vi "Mining and Dumping_r4.vi"() -> ()   [LabVIEW 2015]
uses:
  <vilib>/myRIO/Instrument Drivers/Onboard IO/PWM/typedefs/PWM Reference.ctl
  <vilib>/myRIO/Common/Instrument Driver Framework/Utilities/typedefs/myRIO Generic Hardware Reference.ctl
  <vilib>/myRIO/Common/Instrument Driver Framework/Utilities/typedefs/Hardware Version Enum.ctl
  <vilib>/myRIO/Common/Instrument Driver Framework/Utilities/typedefs/myRIO v1.0 Reference.ctl
  <vilib>/myRIO/Common/Instrument Driver Framework/Utilities/typedefs/Generic FPGA Reference.ctl
  <vilib>/myRIO/Common/Instrument Driver Framework/myRIO v1.0/PWM/typedefs/PWM Channels Enum.ctl
  <vilib>/myRIO/Instrument Drivers/Onboard IO/PWM/typedefs/PWM Configuration.ctl
  <vilib>/userdefined/High Color/nirio_resource_hc.ctl
  <vilib>/myRIO/Instrument Drivers/Onboard IO/AI/typedefs/AI Reference.ctl
  <vilib>/myRIO/Common/Instrument Driver Framework/myRIO v1.0/AI/typedefs/AI Channels List.ctl
  <vilib>/myRIO/Common/Instrument Driver Framework/myRIO v1.0/AI/typedefs/AI Channels Enum.ctl
  <vilib>/myRIO/Common/Instrument Driver Framework/Utilities/typedefs/Analog Scaling Constants List.ctl
  <vilib>/myRIO/Common/Instrument Driver Framework/Utilities/typedefs/Analog Scaling Constants.ctl
  <vilib>/myRIO/Common/Instrument Driver Framework/Utilities/vis/Is FPGA Ref Available.vi
  <vilib>/myRIO/Common/Instrument Driver Framework/myRIO v1.0/PWM/vis/myRIO v1.1 Open PWM.vi
  <vilib>/myRIO/Instrument Drivers/Onboard IO/PWM/vis/Set Duty Cycle and Frequency.vi
  <vilib>/myRIO/Common/Instrument Driver Framework/myRIO v1.0/AI/vis/myRIO v1.1 Open AI.vi
  <vilib>/myRIO/Instrument Drivers/Onboard IO/AI/vis/Read.vi
  <vilib>/myRIO/Common/Instrument Driver Framework/Utilities/vis/Validate Channels.vi
  <vilib>/myRIO/Common/Instrument Driver Framework/myRIO v1.0/PWM/vis/myRIO v1.0 Reserve PWM.vi
  <vilib>/myRIO/Common/Instrument Driver Framework/myRIO v1.0/AI/vis/myRIO v1.0 Reserve AI.vi
  <vilib>/myRIO/Common/Instrument Driver Framework/myRIO v1.0/PWM/vis/myRIO v1.0 Build MUX Configuration PWM.vi
  <vilib>/myRIO/Common/Instrument Driver Framework/myRIO v1.0/Resource Manager/vis/myRIO v1.0 Reserve Channel List.vi
  <vilib>/myRIO/Common/Instrument Driver Framework/myRIO v1.0/AI/vis/myRIO v1.0 Build MUX Configuration AI.vi
  <vilib>/myRIO/Common/Instrument Driver Framework/myRIO v1.0/Resource Manager/vis/myRIO v1.0 Create Configuration List.vi
  <vilib>/myRIO/Common/Instrument Driver Framework/myRIO v1.0/Resource Manager/vis/myRIO v1.0 Reserve Channel.vi
  <vilib>/myRIO/Common/Instrument Driver Framework/myRIO v1.0/Resource Manager/vis/myRIO v1.0 Unreserve Channel.vi
  <vilib>/myRIO/Common/Instrument Driver Framework/myRIO v1.0/Resource Manager/vis/myRIO v1.0 Build Mutex Name.vi
  <vilib>/Utility/VariantDataType/GetNumericInfo.vi
  <vilib>/Utility/error.llb/Error Cluster From Error Code.vi
  <vilib>/myRIO/Common/Instrument Driver Framework/myRIO v1.0/myRIO v1.1 Open.vi
  <vilib>/myRIO/Common/Instrument Driver Framework/Utilities/vis/IO Manager.vi
  <vilib>/myRIO/Common/Instrument Driver Framework/Utilities/vis/Configuration Manager.vi
  <vilib>/myRIO/Common/Instrument Driver Framework/myRIO v1.0/Resource Manager/vis/myRIO v1.0 Configure IO.vi
  <vilib>/myRIO/Common/Instrument Driver Framework/myRIO v1.0/myRIO v1.0 Close.vi
  <vilib>/myRIO/Common/Instrument Driver Framework/myRIO v1.0/PWM/vis/myRIO v1.0 Write PWM.vi
  <vilib>/myRIO/Common/Instrument Driver Framework/myRIO v1.0/AI/vis/myRIO v1.0 Get Scaling Constants AI.vi
  <vilib>/myRIO/Common/Instrument Driver Framework/myRIO v1.0/AI/vis/myRIO v1.0 Read AI.vi
  <vilib>/myRIO/Express VI/Onboard IO/PWM/PWM Express VI.xnode
  <vilib>/myRIO/Instrument Drivers/Onboard IO/PWM/vis/myRIO PWM Open.xnode
  <vilib>/myRIO/Express VI/Onboard IO/AI/AI Express VI.xnode
  <vilib>/myRIO/Instrument Drivers/Onboard IO/AI/vis/myRIO AI Open.xnode
  <vilib>/myRIO/Instrument Drivers/Onboard IO/PWM/PWM.lvlib
  <vilib>/myRIO/Instrument Drivers/Onboard IO/AI/AI.lvlib
panel:
  out "unjammed":bool
  in  "Mine or Dump":i16
  out "Stop Dumping":bool
  in  "Stop":bool
  out "Servo Positioin 2":dbl
  out "Servo Position 1":dbl
  out "Servo Stop":i64
  out "Stop Mining":bool
  out "Full":bool
  # "0=Idle\n1=Mine\n-1=Dump"
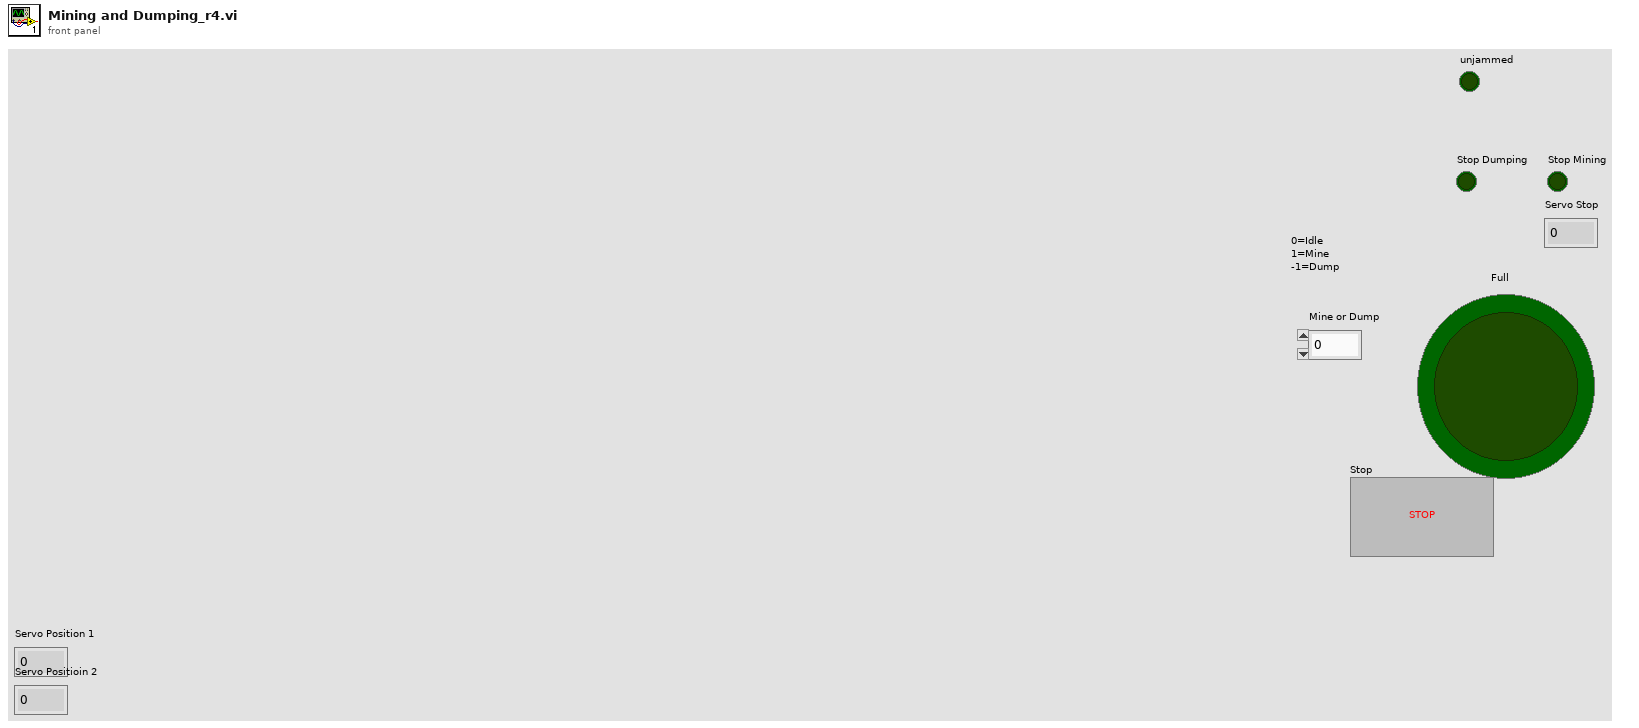
[diagram p1: front panel]
types:
  T1 = typedef "PWM.lvlib/PWM Reference.ctl" = cluster{"myRIO Reference":T2, "PWM Channels Enum":T6, "PWM Configuration":T7}
  T2 = typedef "myRIO Generic Hardware Reference.ctl" = cluster{"myRIO Model":T3, "myRIO Hardware Reference":T4}
  T3 = typedef "Hardware Version Enum.ctl" = enum16{"Unknown", "myRIO-1900", "myRIO-1950", "roboRIO"}
  T4 = typedef "myRIO v1.0 Reference.ctl" = cluster{"Generic FPGA Reference":T5, "Allow multiple opens":bool}
  T5 = typedef "Generic FPGA Reference.ctl" = refnum<k20>
  T6 = typedef "PWM Channels Enum.ctl" = enum16{"Not Connected", "C/PWM0", "C/PWM1", "A/PWM0", "A/PWM1", "A/PWM2", "B/PWM0", "B/PWM1", "B/PWM2", "PWM/PWM0", "PWM/PWM1", "PWM/PWM2", "PWM/PWM3", "PWM/PWM4", "PWM/PWM5", "PWM/PWM6", "PWM/PWM7", "PWM/PWM8", "PWM/PWM9"}
  T7 = typedef "PWM.lvlib/PWM Configuration.ctl" = cluster{"Frequency":dbl, "Duty Cycle":dbl}
  T8 = typedef "nirio_resource_hc.ctl" = tag
  T9 = typedef "AI.lvlib/AI Reference.ctl" = cluster{"myRIO Reference":T2, "AI Channels List":T10, "AI Scaling Constants List":T12}
  T10 = typedef "AI Channels List.ctl" = T11[]
  T11 = typedef "AI Channels Enum.ctl" = enum16{"Not Connected", "AudioIn/Left", "AudioIn/Right", "C/AI0", "C/AI1", "A/AI0", "A/AI1", "A/AI2", "A/AI3", "B/AI0", "B/AI1", "B/AI2", "B/AI3", "AI/AI0", "AI/AI1", "AI/AI2", "AI/AI3"}
  T12 = typedef "Analog Scaling Constants List.ctl" = T13[]
  T13 = typedef "Analog Scaling Constants.ctl" = cluster{"LSB Weight (Volts)":dbl, "Offset (Volts)":dbl, "Signed?":bool}
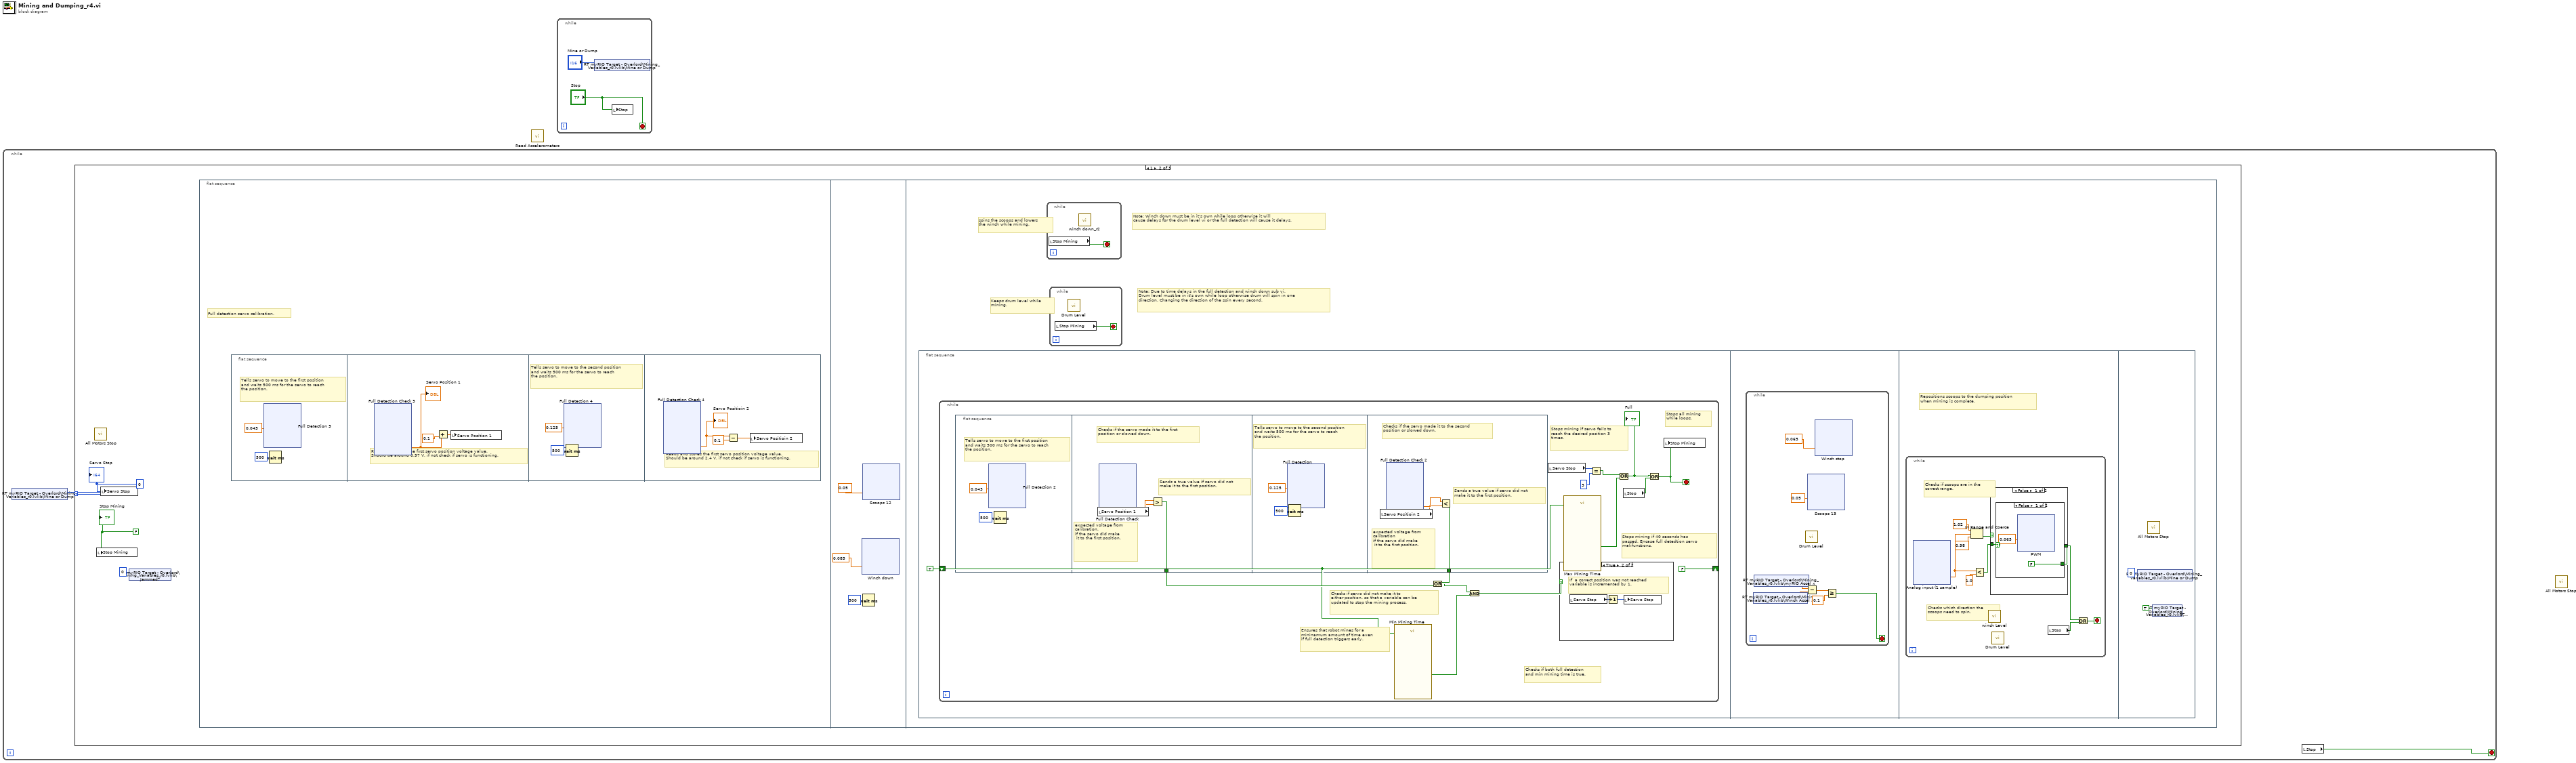
[diagram p0: block diagram]
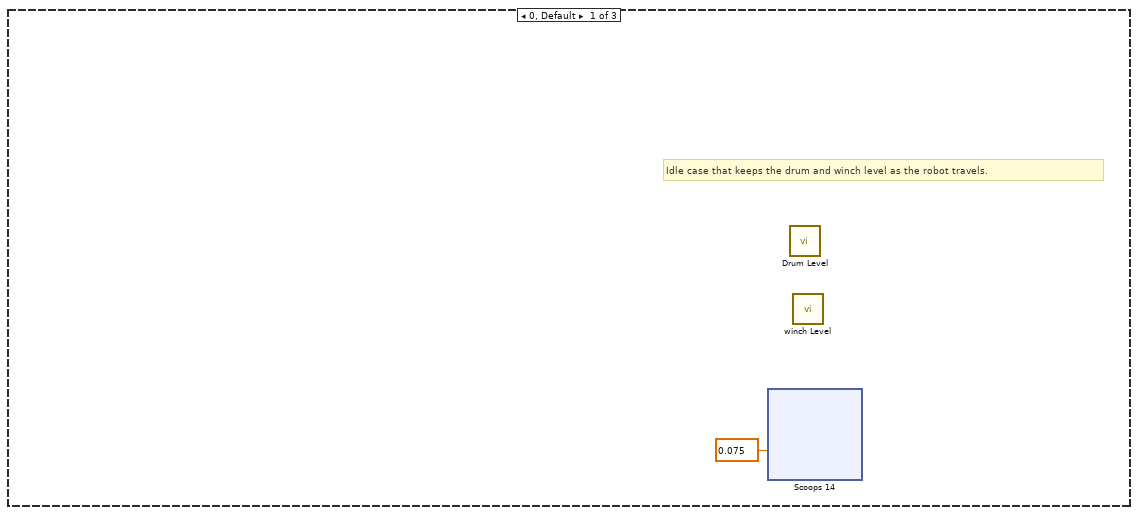
[diagram p2: hidden frame]
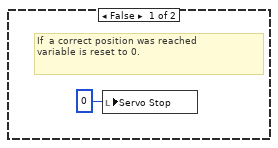
[diagram p3: hidden frame]
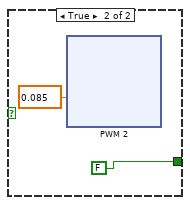
[diagram p4: hidden frame]
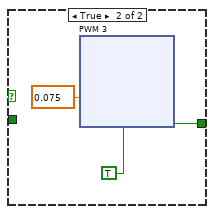
[diagram p5: hidden frame]
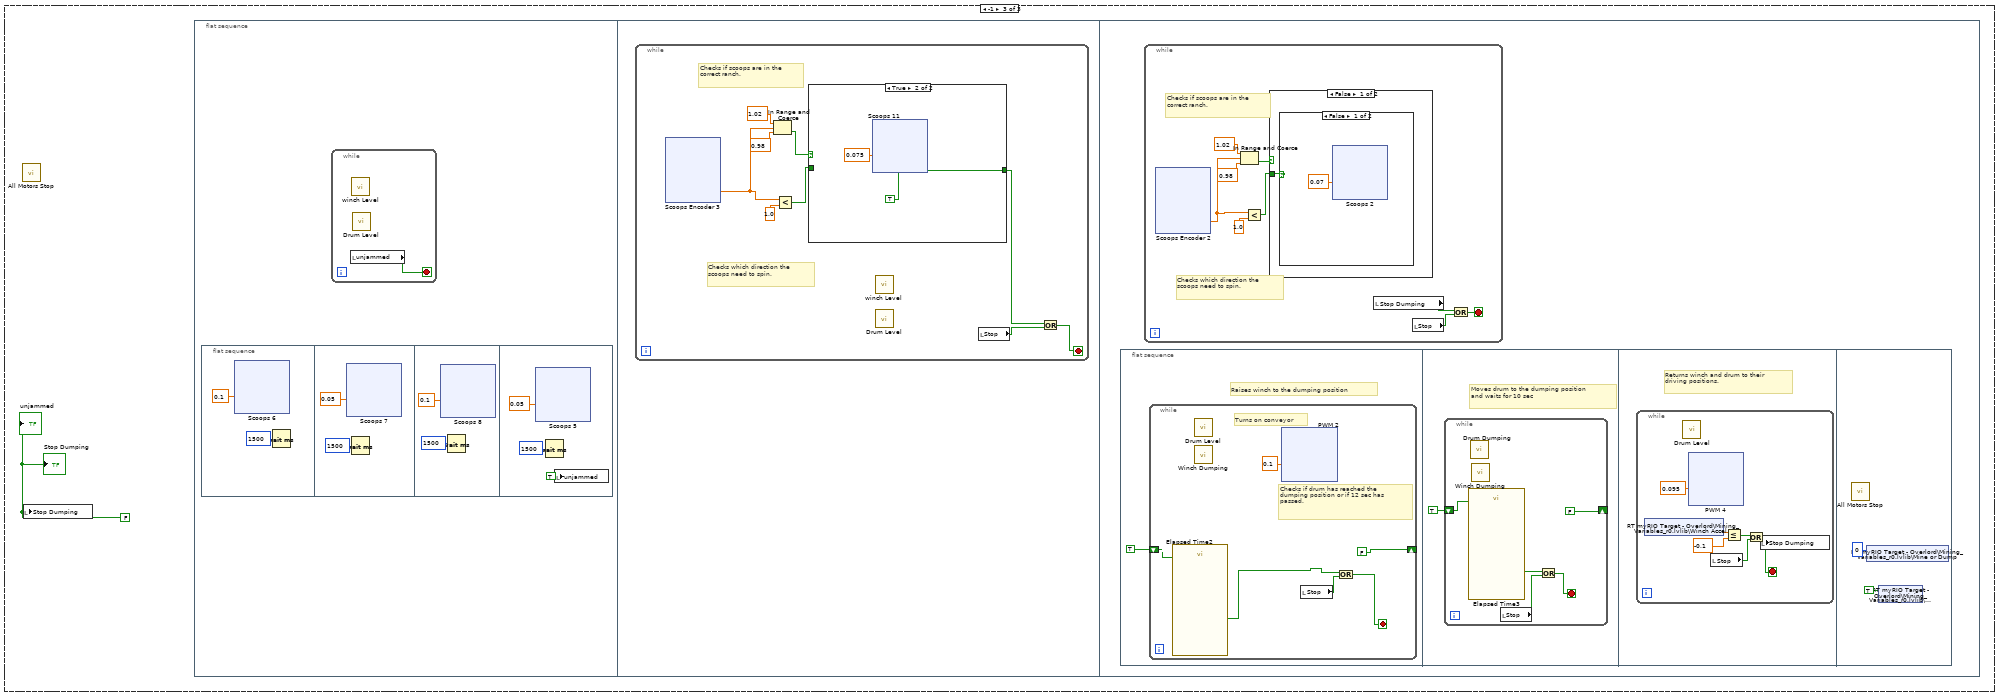
[diagram p6: hidden frame]
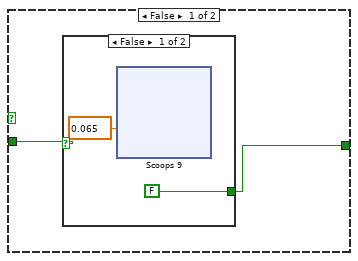
[diagram p7: hidden frame]
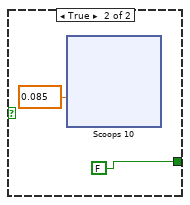
[diagram p8: hidden frame]
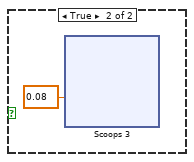
[diagram p9: hidden frame]
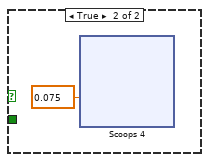
[diagram p10: hidden frame]
diagram:
  n1 = while {
    stop <- w1 stop-if-true
    n2 = shared-variable "RT myRIO Target - Overlord\\Mining_Variables_r0.lvlib\\Mine or Dump"() -> (w2:i16)  [unwired: 1 in, 1 out]
    n3 = case shown="1" w2 {
      frame 0, Default {
        # "Idle case that keeps the drum and winch level as the robot travels."
        n4 = xnode "Scoops 14"("Duty Cycle"=0.075) -> ()  [unwired: 1 in, 1 out]
        n5 = call "Drum Level.vi"() -> ()  [unwired: 12 in]
        n6 = call "winch Level.vi"() -> ()  [unwired: 12 in]
      }
      frame 1 {
        w41 = FALSE ("Stop")
        w40 = i64 0 ("Servo Stop")
        n7 = call "All Motors Stop.vi"() -> ()  [unwired: 12 in]
        n8 = local write "Stop Mining"(w41) -> ()
        n9 = local write "Servo Stop"(w40) -> ()
        n10 = shared-variable "RT myRIO Target - Overlord\\Mining_Variables_r0.lvlib\\Jammed?"(u16 0 ("Jammed?")) -> ()  [unwired: 1 in, 1 out]
        n11 = flat-sequence {
          frame #0 {
            # "Full detection servo calibration."
            n12 = flat-sequence {
              frame #0 {
                # "Tells servo to move to the first position\nand waits 500 ms for the servo to reach \nthe position."
                n13 = xnode "Full Detection 3"("Duty Cycle"=0.043) -> ()  [unwired: 1 in, 1 out]
                n14 = Wait (ms)(milliseconds to wait=u32 500) -> ()  [unwired: 1 out]
              }
              frame #1 {
                # "Reads and stores the first servo position voltage value. \nShould be around 0.97 V. if not check if servo is functioning."
                n15 = xnode "Full Detection Check 3"() -> ("A/AI0 (Pin 3)"=w80:dbl)  [unwired: 1 in, 1 out]
                "Servo Position 1" <- w80
                n16 = Add(x=w80, y=0.1) -> (x+y=w81:dbl)
                n17 = local write "Servo Position 1"(w81) -> ()
              }
              frame #2 {
                # "Tells servo to move to the second position\nand waits 500 ms for the servo to reach \nthe position."
                n18 = xnode "Full Detection 4"("Duty Cycle"=0.125) -> ()  [unwired: 1 in, 1 out]
                n19 = Wait (ms)(milliseconds to wait=u32 500) -> ()  [unwired: 1 out]
              }
              frame #3 {
                # "Reads and stores the first servo position voltage value. \nShould be around 2.4 V. if not check if servo is functioning."
                n20 = xnode "Full Detection Check 4"() -> ("A/AI0 (Pin 3)"=w157:dbl)  [unwired: 1 in, 1 out]
                "Servo Positioin 2" <- w157
                n21 = Subtract(x=w157, y=0.1) -> (x-y=w158:dbl)
                n22 = local write "Servo Positioin 2"(w158) -> ()
              }
            }
          }
          frame #1 {
            n23 = xnode "Winch down"("Duty Cycle"=0.085) -> ()  [unwired: 1 in, 1 out]
            n24 = xnode "Scoops 12"("Duty Cycle"=0.05) -> ()  [unwired: 1 in, 1 out]
            n25 = Wait (ms)(milliseconds to wait=u32 500) -> ()  [unwired: 1 out]
          }
          frame #2 {
            # "Note: Winch down must be in it's own while loop otherwise it will \ncause delays for the drum level vi or the full detection will cause it delays."
            # "Note: Due to time delays in the full detection and winch down sub vi.\nDrum level must be in it's own while loop otherwise drum will spin in one\ndirection. Changing the direction of the spin every second."
            # "spins the scoops and lowers\nthe winch while mining."
            # "Keeps drum level while \nmining."
            n26 = flat-sequence {
              frame #0 {
                n27 = while {
                  shift-right: [FALSE] -> _
                  shift-left: TRUE -> [w271]
                  stop <- w274 stop-if-true
                  # "Stops all mining \nwhile loops."
                  # "Stops mining if 40 seconds has \npassed. Encase full detedtion servo \nmalifunctions."
                  # "Stops mining if servo fails to \nreach the desired position 3\ntimes."
                  # "Checks if both full detection \nand min mining time is true."
                  # "Ensures that robot mines for a \nmininamum amount of time even\nif full detection triggers early."
                  # "Checks if servo did not make it to\neither position. so that a variable can be \nupdated to stop the mining process."
                  n28 = flat-sequence {
                    tunnel: [w327] -> w283
                    tunnel: [w403] -> w284
                    frame #0 {
                      # "Tells servo to move to the first position\nand waits 500 ms for the servo to reach \nthe position."
                      n29 = xnode "Full Detection 2"("Duty Cycle"=0.043) -> ()  [unwired: 1 in, 1 out]
                      n30 = Wait (ms)(milliseconds to wait=u32 500) -> ()  [unwired: 1 out]
                    }
                    frame #1 {
                      # "Sends a true value if servo did not \nmake it to the first position."
                      # "expected voltage from \ncalibration.\nif the servo did make\n it to the first position."
                      # "Checks if the servo made it to the first \nposition or slowed down."
                      n31 = local read "Servo Position 1"() -> (w325:dbl)
                      n32 = xnode "Full Detection Check"() -> ("A/AI0 (Pin 3)"=w326:dbl)  [unwired: 1 in, 1 out]
                      n33 = Greater?(x=w326, y=w325) -> (0:w327:bool)
                    }
                    frame #2 {
                      # "Tells servo to move to the second position\nand waits 500 ms for the servo to reach \nthe position."
                      n34 = xnode "Full Detection"("Duty Cycle"=0.125) -> ()  [unwired: 1 in, 1 out]
                      n35 = Wait (ms)(milliseconds to wait=u32 500) -> ()  [unwired: 1 out]
                    }
                    frame #3 {
                      # "Sends a true value if servo did not \nmake it to the first position."
                      # "expected voltage from \ncalibration\nif the servo did make\n it to the first position."
                      # "Checks if the servo made it to the second \nposition or slowed down."
                      n36 = local read "Servo Positioin 2"() -> (w402:dbl)
                      n37 = xnode "Full Detection Check 2"() -> ("A/AI0 (Pin 3)"=w404:dbl)  [unwired: 1 in, 1 out]
                      n38 = Less?(x=w404, y=w402) -> (x < y?=w403:bool)
                    }
                  }
                  n39 = call "Min Mining Time"("Reset"=w271) -> ("Time has Elapsed"=w276:bool)  [unwired: 11 in, 7 out]
                  n40 = Or(x=w284, y=w283) -> (x .or. y?=w277:bool)
                  n41 = And(x=w277, y=w276) -> (x .and. y?=w278:bool)
                  n42 = local read "Servo Stop"() -> (w281:i64)
                  n43 = case shown="True" w278 {
                    frame False {
                      # "If  a correct position was reached \nvariable is reset to 0."
                      n44 = local write "Servo Stop"(i64 0 ("Servo Stop")) -> ()
                    }
                    frame True {
                      # "If  a correct position was not reached \nvariable is incremented by 1."
                      n45 = local read "Servo Stop"() -> (w287:i64)
                      n46 = Increment(x=w287) -> (x+1=w286:i64)
                      n47 = local write "Servo Stop"(w286) -> ()
                    }
                  }
                  n48 = call "Max Mining Time"("Reset"=w271) -> ("Time has Elapsed"=w280:bool)  [unwired: 11 in, 7 out]
                  n49 = Equal?(x=w281, y=i64 3) -> (x = y?=w279:bool)
                  n50 = Or(x=w279, y=w280) -> (x .or. y?=w275:bool)
                  "Full" <- w275
                  n51 = local read "Stop"() -> (w273:bool)
                  n52 = Or(x=w275, y=w273) -> (x .or. y?=w274:bool)
                  n53 = local write "Stop Mining"(w274) -> ()
                }
              }
              frame #1 {
                n54 = while {
                  stop <- w442 stop-if-true
                  n55 = shared-variable "RT myRIO Target - Overlord\\Mining_Variables_r0.lvlib\\Winch Accel x"() -> (w445:dbl)  [unwired: 1 in, 1 out]
                  n56 = shared-variable "RT myRIO Target - Overlord\\Mining_Variables_r0.lvlib\\myRIO Accel x"() -> (w446:dbl)  [unwired: 1 in, 1 out]
                  n57 = call "Drum Level.vi"() -> ()  [unwired: 12 in]
                  n58 = Subtract(x=w446, y=w445) -> (x-y=w444:dbl)
                  n59 = xnode "Scoops 13"("Duty Cycle"=0.05) -> ()  [unwired: 1 in, 1 out]
                  n60 = xnode "Winch stop"("Duty Cycle"=0.065) -> ()  [unwired: 1 in, 1 out]
                  n61 = Greater Or Equal?(x=w444, y=0.1) -> (x >= y?=w442:bool)
                }
              }
              frame #2 {
                # "Repositions scoops to the dumping position\nwhen mining is complete."
                n62 = while {
                  stop <- w521 stop-if-true
                  # "Checks which direction the \nscoops need to spin."
                  # "Checks if scoops are in the\ncorrect range."
                  n63 = xnode "Analog input (1 sample)"() -> ("A/AI1 (Pin 5)"=w524:dbl)  [unwired: 1 in, 1 out]
                  n64 = In Range and Coerce(upper limit=1.02, x=w524, lower limit=0.98) -> (In Range?=w525:bool)  [unwired: 1 out]
                  n65 = Less?(x=w524, y=1.0) -> (x < y?=w526:bool)
                  n66 = call "winch Level.vi"() -> ()  [unwired: 12 in]
                  n67 = case shown="False" w525 {
                    tunnel: w526 -> [w529 _]
                    tunnel: [w528 TRUE] -> w520
                    frame False {
                      n68 = case shown="False" w529 {
                        tunnel: [FALSE FALSE] -> w528
                        frame False {
                          n69 = xnode "PWM"("Duty Cycle"=0.065) -> ()  [unwired: 1 in, 1 out]
                        }
                        frame True {
                          n70 = xnode "PWM 2"("Duty Cycle"=0.085) -> ()  [unwired: 1 in, 1 out]
                        }
                      }
                    }
                    frame True {
                      n71 = xnode "PWM 3"("Duty Cycle"=0.075) -> ()  [unwired: 1 in, 1 out]
                    }
                  }
                  n72 = call "Drum Level.vi"() -> ()  [unwired: 12 in]
                  n73 = local read "Stop"() -> (w519:bool)
                  n74 = Or(x=w520, y=w519) -> (x .or. y?=w521:bool)
                }
              }
              frame #3 {
                n75 = shared-variable "RT myRIO Target - Overlord\\Mining_Variables_r0.lvlib\\Mine or Dump"(i16 0 ("Mine or Dump")) -> ()  [unwired: 1 in, 1 out]
                n76 = call "All Motors Stop.vi"() -> ()  [unwired: 12 in]
                n77 = shared-variable "RT myRIO Target - Overlord\\Mining_Variables_r0.lvlib\\Stop"(TRUE ("Stop")) -> ()  [unwired: 1 in, 1 out]
              }
            }
            n78 = while {
              stop <- w269 stop-if-true
              n79 = local read "Stop Mining"() -> (w269:bool)
              n80 = call "winch down_r2.vi"() -> ()  [unwired: 12 in]
            }
            n81 = while {
              stop <- w680 stop-if-true
              n82 = local read "Stop Mining"() -> (w680:bool)
              n83 = call "Drum Level.vi"() -> ()  [unwired: 12 in]
            }
          }
        }
        "Stop Mining" <- w41
        "Servo Stop" <- w40
      }
      frame -1 {
        w681 = FALSE
        n84 = call "All Motors Stop.vi"() -> ()  [unwired: 12 in]
        n85 = local write "Stop Dumping"(w681) -> ()
        n86 = flat-sequence {
          frame #0 {
            n87 = flat-sequence {
              frame #0 {
                n88 = xnode "Scoops 6"("Duty Cycle"=0.1) -> ()  [unwired: 1 in, 1 out]
                n89 = Wait (ms)(milliseconds to wait=u32 1500) -> ()  [unwired: 1 out]
              }
              frame #1 {
                n90 = xnode "Scoops 7"("Duty Cycle"=0.05) -> ()  [unwired: 1 in, 1 out]
                n91 = Wait (ms)(milliseconds to wait=u32 1500) -> ()  [unwired: 1 out]
              }
              frame #2 {
                n92 = xnode "Scoops 8"("Duty Cycle"=0.1) -> ()  [unwired: 1 in, 1 out]
                n93 = Wait (ms)(milliseconds to wait=u32 1500) -> ()  [unwired: 1 out]
              }
              frame #3 {
                n94 = xnode "Scoops 5"("Duty Cycle"=0.05) -> ()  [unwired: 1 in, 1 out]
                n95 = Wait (ms)(milliseconds to wait=u32 1500) -> ()  [unwired: 1 out]
                n96 = local write "unjammed"(TRUE ("unjammed")) -> ()
              }
            }
            n97 = while {
              stop <- w682 stop-if-true
              n98 = local read "unjammed"() -> (w682:bool)
              n99 = call "winch Level.vi"() -> ()  [unwired: 12 in]
              n100 = call "Drum Level.vi"() -> ()  [unwired: 12 in]
            }
          }
          frame #1 {
            n101 = while {
              stop <- w834 stop-if-true
              # "Checks which direction the \nscoops need to spin."
              # "Checks if scoops are in the\ncorrect ranch."
              n102 = xnode "Scoops Encoder 3"() -> ("A/AI1 (Pin 5)"=w837:dbl)  [unwired: 1 in, 1 out]
              n103 = In Range and Coerce(upper limit=1.02, x=w837, lower limit=0.98) -> (In Range?=w836:bool)  [unwired: 1 out]
              n104 = Less?(x=w837, y=1.0) -> (x < y?=w835:bool)
              n105 = case shown="True" w836 {
                tunnel: w835 -> [w842 _]
                tunnel: [w841 TRUE] -> w833
                frame False {
                  n106 = case shown="False" w842 {
                    tunnel: [FALSE FALSE] -> w841
                    frame False {
                      n107 = xnode "Scoops 9"("Duty Cycle"=0.065) -> ()  [unwired: 1 in, 1 out]
                    }
                    frame True {
                      n108 = xnode "Scoops 10"("Duty Cycle"=0.085) -> ()  [unwired: 1 in, 1 out]
                    }
                  }
                }
                frame True {
                  n109 = xnode "Scoops 11"("Duty Cycle"=0.075) -> ()  [unwired: 1 in, 1 out]
                }
              }
              n110 = call "winch Level.vi"() -> ()  [unwired: 12 in]
              n111 = call "Drum Level.vi"() -> ()  [unwired: 12 in]
              n112 = local read "Stop"() -> (w832:bool)
              n113 = Or(x=w833, y=w832) -> (x .or. y?=w834:bool)
            }
          }
          frame #2 {
            n114 = flat-sequence {
              frame #0 {
                # "Raises winch to the dumping position"
                n115 = while {
                  shift-right: [FALSE ("Reset")] -> _
                  shift-left: TRUE ("Reset") -> [w1148]
                  stop <- w1151 stop-if-true
                  # "Turns on conveyor"
                  # "Checks if drum has reached the \ndumping position or if 12 sec has \npassed."
                  n116 = call "Elapsed Time2"("Reset"=w1148) -> ("Time has Elapsed"=w1147:bool)  [unwired: 11 in, 7 out]
                  n117 = call "Drum Level.vi"() -> ()  [unwired: 12 in]
                  n118 = call "Winch Dumping.vi"() -> ()  [unwired: 12 in]
                  n119 = xnode "PWM 2"("Duty Cycle"=0.1) -> ()  [unwired: 1 in, 1 out]
                  n120 = local read "Stop"() -> (w1150:bool)
                  n121 = Or(x=w1147, y=w1150) -> (x .or. y?=w1151:bool)
                }
              }
              frame #1 {
                # "Moves drum to the dumping position\nand waits for 10 sec"
                n122 = while {
                  shift-right: [FALSE ("Reset")] -> _
                  shift-left: TRUE ("Reset") -> [w1189]
                  stop <- w1193 stop-if-true
                  n123 = call "Elapsed Time3"("Reset"=w1189) -> ("Time has Elapsed"=w1192:bool)  [unwired: 11 in, 7 out]
                  n124 = call "Drum Dumping.vi"() -> ()  [unwired: 12 in]
                  n125 = call "Winch Dumping.vi"() -> ()  [unwired: 12 in]
                  n126 = local read "Stop"() -> (w1191:bool)
                  n127 = Or(x=w1192, y=w1191) -> (x .or. y?=w1193:bool)
                }
              }
              frame #2 {
                # "Returns winch and drum to their \ndriving positions."
                n128 = while {
                  stop <- w1194 stop-if-true
                  n129 = shared-variable "RT myRIO Target - Overlord\\Mining_Variables_r0.lvlib\\Winch Accel x"() -> (w1199:dbl)  [unwired: 1 in, 1 out]
                  n130 = call "Drum Level.vi"() -> ()  [unwired: 12 in]
                  n131 = xnode "PWM 4"("Duty Cycle"=0.095) -> ()  [unwired: 1 in, 1 out]
                  n132 = local read "Stop"() -> (w1195:bool)
                  n133 = Less Or Equal?(x=w1199, y=-0.1) -> (x <= y?=w1196:bool)
                  n134 = Or(x=w1196, y=w1195) -> (x .or. y?=w1194:bool)
                  n135 = local write "Stop Dumping"(w1194) -> ()
                }
              }
              frame #3 {
                n136 = call "All Motors Stop.vi"() -> ()  [unwired: 12 in]
                n137 = shared-variable "RT myRIO Target - Overlord\\Mining_Variables_r0.lvlib\\Mine or Dump"(i16 0 ("Mine or Dump")) -> ()  [unwired: 1 in, 1 out]
                n138 = shared-variable "RT myRIO Target - Overlord\\Mining_Variables_r0.lvlib\\Stop"(TRUE ("Stop")) -> ()  [unwired: 1 in, 1 out]
              }
            }
            n139 = while {
              stop <- w993 stop-if-true
              # "Checks which direction the \nscoops need to spin."
              # "Checks if scoops are in the\ncorrect ranch."
              n140 = xnode "Scoops Encoder 2"() -> ("A/AI1 (Pin 5)"=w996:dbl)  [unwired: 1 in, 1 out]
              n141 = In Range and Coerce(upper limit=1.02, x=w996, lower limit=0.98) -> (In Range?=w997:bool)  [unwired: 1 out]
              n142 = Less?(x=w996, y=1.0) -> (x < y?=w998:bool)
              n143 = case shown="False" w997 {
                tunnel: w998 -> [w1000 _]
                frame False {
                  n144 = case shown="False" w1000 {
                    frame False {
                      n145 = xnode "Scoops 2"("Duty Cycle"=0.07) -> ()  [unwired: 1 in, 1 out]
                    }
                    frame True {
                      n146 = xnode "Scoops 3"("Duty Cycle"=0.08) -> ()  [unwired: 1 in, 1 out]
                    }
                  }
                }
                frame True {
                  n147 = xnode "Scoops 4"("Duty Cycle"=0.075) -> ()  [unwired: 1 in, 1 out]
                }
              }
              n148 = local read "Stop Dumping"() -> (w991:bool)
              n149 = local read "Stop"() -> (w992:bool)
              n150 = Or(x=w991, y=w992) -> (x .or. y?=w993:bool)
            }
          }
        }
        "Stop Dumping" <- w681
        "unjammed" <- w681
      }
    }
    n151 = local read "Stop"() -> (w1:bool)
  }
  n152 = call "Read Accelerometers.vi"() -> ()  [unwired: 11 in, 9 out]
  n153 = while {
    stop <- "Stop" stop-if-true
    n154 = shared-variable "RT myRIO Target - Overlord\\Mining_Variables_r0.lvlib\\Mine or Dump"("Mine or Dump") -> ()  [unwired: 1 in, 1 out]
    n155 = local write "Stop"("Stop") -> ()
  }
  n156 = call "All Motors Stop.vi"() -> ()  [unwired: 12 in]
